vi "Ctrl.ListBox.StyleFont.vi"(8 "error in (no error)":errorcluster, 10 "Font Info":T1, 11 "Listbox Ref":refnum<vi>) -> (0 "error out":errorcluster, 3 "Listbox Ref out":refnum<vi>)   [LabVIEW 2017, in "JKI Simple Localization.lvlib"]
uses:
  API/JKI Simple Localization.lvlib
  Definitions/Private/Font Info.ctl
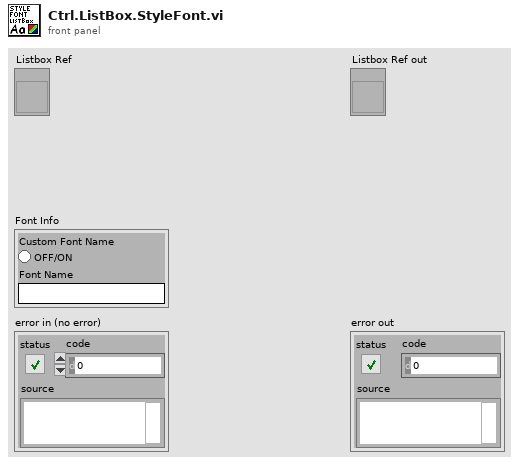
[diagram p1: front panel]
types:
  T1 = typedef "JKI Simple Localization.lvlib/Font Info.ctl" = cluster{"Custom Font Name":bool, "Font Name":string}
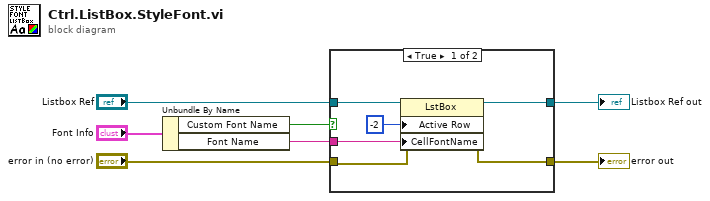
[diagram p0: block diagram]
diagram:
  n1 = Unbundle By Name("Font Info") -> ("Custom Font Name"=w6:bool, "Font Name"=w3:string)
  n2 = case shown="True" w6 {
    tunnel: [w8 w15] -> w5
    tunnel: "error in (no error)" -> [w9 w15]
    tunnel: w3 -> [w12 _]
    tunnel: "Listbox Ref" -> [w11 w14]
    tunnel: [w10 w14] -> w1
    frame True {
      n3 = property class="LstBox"(reference=w11, error in=w9, "Active Row"=-2 ("Active Row:Active Row Number"), "CellFontName"=w12) -> (reference out=w10:refnum<vi>, error out=w8:errorcluster)
    }
    frame False {
    }
  }
  "error out" <- w5
  "Listbox Ref out" <- w1
